vi "cw_4_1.vi"() -> ()   [LabVIEW 2022 SP3]
uses:
  3cdbe356-b82f-4c40-9c51-a14b2e5d92a4.vi
  33fc5f7e-09e9-4883-9bc9-fae40cb30b02.vi
  <vilib>/Array/Sort 2D Array - Pop Stack.vi
  <vilib>/Array/Sort 2D Array - Push Stack.vi
  3cdbe356-b82f-4c40-9c51-a14b2e5d92a4.vi/269d4b3b-47f5-49e3-8884-44851e4dd9d5.vi
  3cdbe356-b82f-4c40-9c51-a14b2e5d92a4.vi/6d99389c-673d-4efb-bf33-19b32bcf4cf8.vi
  33fc5f7e-09e9-4883-9bc9-fae40cb30b02.vi/269d4b3b-47f5-49e3-8884-44851e4dd9d5.vi
  33fc5f7e-09e9-4883-9bc9-fae40cb30b02.vi/6d99389c-673d-4efb-bf33-19b32bcf4cf8.vi
panel:
  out "Array 2":dbl[][](array[numeric])
  in  "Array":dbl[][](array[numeric])
  in  "Select column":i32
  in  "Select row":i32
  in  "Sort by:":enum16{"Column", "Row"}(ring)
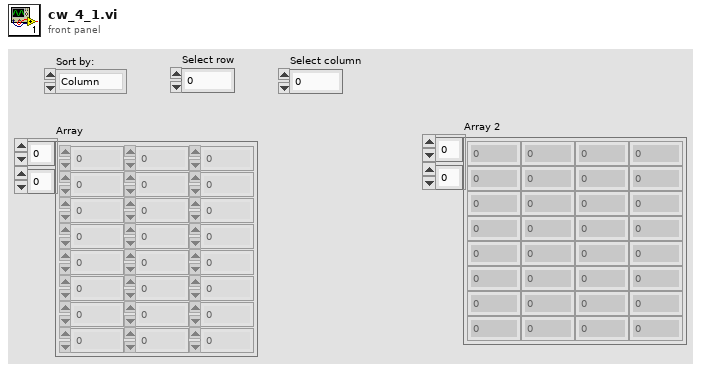
[diagram p1: front panel]
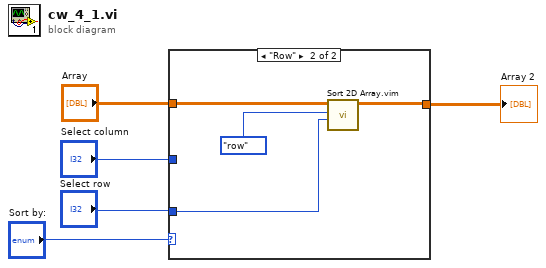
[diagram p0: block diagram]
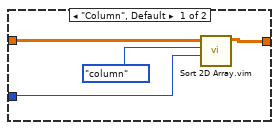
[diagram p2: hidden frame]
diagram:
  n1 = case shown="\"Row\"" "Sort by:" {
    tunnel: "Select column" -> [w6 _]
    tunnel: "Select row" -> [_ w12]
    tunnel: "Array" -> [w8 w13]
    tunnel: [w7 w11] -> w1
    frame "Column", Default {
      n2 = call "Sort 2D Array.vim"("index"=w6, "dimension to index (column)"=enum16{"column", "row"}."column", "2D array"=w8) -> ("sorted 2D array"=w7:dbl[][])  [unwired: 7 in, 1 out]
    }
    frame "Row" {
      n3 = call "Sort 2D Array.vim"("index"=w12, "dimension to index (column)"=enum16{"column", "row"}."row", "2D array"=w13) -> ("sorted 2D array"=w11:dbl[][])  [unwired: 7 in, 1 out]
    }
  }
  "Array 2" <- w1
